vi "checkBeginEnemyPossesionAtOurField.vi"(8 "error in (no error)":errorcluster, 10 "Game":refnum<class "Game.lvclass">, 11 "EnemyPossessionAtOurFieldPlay in":refnum<class "EnemyPossessionAtOurFieldPlay.lvclass">) -> (0 "error out":errorcluster, 2 "Begin?":bool, 3 "EnemyPossessionAtOurFieldPlay out":refnum<class "EnemyPossessionAtOurFieldPlay.lvclass">)   [LabVIEW 2023, in "EnemyPossessionAtOurFieldPlay.lvclass"]
uses:
  EnemyPossessionAtOurFieldPlay.lvclass
  Game_class/Game.lvclass
  Team_class/OffensivePlay.ctl
  Referee_class/command_interpreted.ctl
  Events_class/Possession.ctl
  Game_class/Game.lvclass/Game.ctl
  Referee_class/Referee.lvclass/Referee.ctl
  Team_class/Team.lvclass/Team.ctl
  Parameters_class/Parameters.lvclass/Parameters.ctl
  Object_class/Object.lvclass/Object.ctl
  Ball_class/Ball.lvclass/Ball.ctl
  Events_class/Events.lvclass/Events.ctl
  Game_class/Read Referee.vi
  Game_class/Read EventsRef.vi
  Game_class/Read BallRef.vi
  Game_class/Read OffensiveTeam.vi
  Game_class/Read EnemyRef.vi
  Game_class/Read NewParameters.vi
  Game_class/Read FieldRef.vi
  Game_class/Read Parameters.lvclass.vi
  Parameters_class/Read BallVelToAbortPass.vi
  Team_class/Read RobotRef.vi
  Team_class/Read OffensivePlay.vi
  Object_class/Read x.vi
  Ball_class/Read velocityNorm.vi
  Events_class/Read id_touch.vi
  Events_class/Read touch.vi
  Referee_class/Read command_interpreted.vi
  <vilib>/Analysis/_algsub.llb/Vector Norm.vi
  <vilib>/Analysis/_algsub.llb/Real Vector Norm.vi
  Ally_class/Ally.lvclass
  C:/Users/ebert/Documents/codes/SSL/repo/SSL_AI/Team_class/Team.lvclass
  Enemy_class/Enemy.lvclass
  Ball_class/Ball.lvclass
  C:/Users/ebert/Documents/codes/SSL/repo/SSL_AI/Object_class/Object.lvclass
  Referee_class/Referee.lvclass
  Events_class/Events.lvclass
  Field_class/Field.lvclass
  Parameters_class/Parameters.lvclass
  Robot_class/Robot.lvclass
  Utilities_class/Utilities.lvclass
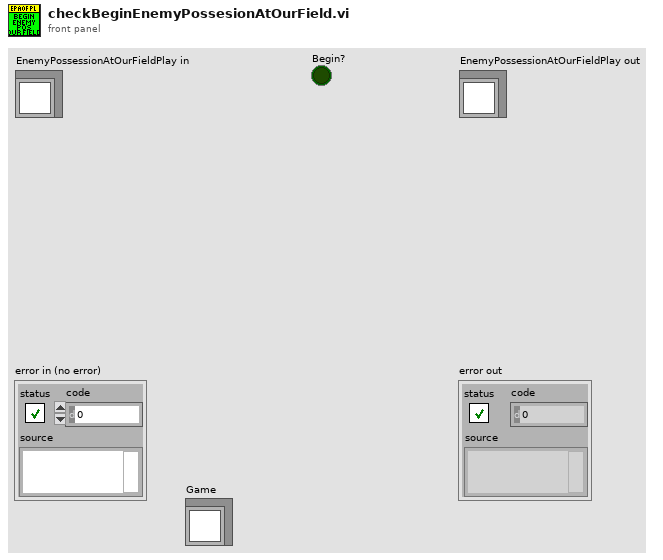
[diagram p1: front panel]
types:
  T1 = typedef "Events.lvclass/Possession.ctl" = enum16{"OurPossession", "TheirPossession", "Contended", "Loose"}
  T2 = typedef "OffensivePlay.ctl" = enum16{"5RobotsPassGamePlay", "5PreparePassGame", "5RobotsKeeperGame", "KeeperPassToStriker", "5RobotsNormalGamePlay", "PrepareKeeperPass", "ACBPass", "ABCPass", "PrepareTriplePass", "TableWithStriker", "TableWith2ndStrikerPlay", "PrepareDoublePass", "PrepareRollToPass", "SimplePass", "PreparePass", "PassToStriker", "BallOutOfField", "PassTo2ndStriker", "StopOffensive", "Prepare Penalty Enemy", "EnemyPossessionAtEnemyField", "EnemyPossesionAtOurField", "TestPlay", "PreparePenaltyAlly", "KickPenaltyAlly", "PrepareKickoffAlly", "PrepareKickoffEnemy", "IndirectEnemy", "DirectEnemy", "PreparePassInGame1", "NormalGame", "DirectKick", "Pass", "Halt", "Timeout", "PassPlay", "PenaltyEnemy"}
  T3 = typedef "command_interpreted.ctl" = enum16{"Goal Ally", "Goal Enemy", "Ball Placement Enemy", "Ball Placement Ally", "Normal Half Time", "Extra Time  Break", "Extra Half Time", "None", "Post Game", "PKA Normal Start", "Prepare Kickoff Ally", "PKE Normal Start", "Prepare Kickoff Enemy", "Force Start", "Halt", "Timeout", "Prepare Penalty Ally", "Prepare Penalty Enemy", "PPA NormalStart", "PPE Normal Start", "Indirect Free Ally", "Direct Free Enemy", "Direct Free Ally", "Indirect Free Enemy", "Stop"}
  T4 = typedef "NewParameters.ctl" = cluster{"PenaltyDistance":dbl, "DistanceAttackerToBackBall":dbl, "Division":enum16{"Div B", "Div A"}, "DistanceToAvoidyEnemyRobot":dbl, "BallPlacementDistance":dbl, "DisatanceBehindBallToStealBall":dbl, "MaxDistanceToPositionKickoff":dbl, "BlockEnemyTarget":bool, "MaxStopVAng":dbl, "DistanceMarkerToEnemy":dbl, "IgnoreDribblerContact":bool, "DistanceToBeginEnemyPosession":dbl, "GoToBallWhenEnemyNotMoving":bool, "EnemyDistanceToReduceVelocity":dbl, "TurnOnEnemyDistanceToReduceVelocity":bool, "EnemyDistanceToShootOutBall":dbl, "DefenseKickBall":bool, "MoreKickToGoal? (0-0.3)":dbl, "ChipKickInEnemyField":bool, "ShootOutRobotId":dbl, "FieldLenghtDenominatorInShootOut":dbl, "AdjustPositionInBallPlacement":bool, "PowerGodPass":dbl, "VelocityAbortEnemyPos":dbl, "MaxDistToBeginPass":dbl, "MinDistToBeginPass":dbl, "VelocityInDirects":dbl, "BadDribblerIDs":i32[], "NewKickToDistanceAroundBall":dbl, "PowerAvoidColisionMarker":dbl, "DistanceToAvoidColisionMarker":dbl, "AvoidBallKick":dbl, "DistanceTryKick":dbl, "SuicideKickDIstance":dbl, "FirstKickAtck":bool, "AdjustFirstKickDistance":dbl, "FirstKickDefense":bool, "AvoidAimLessKick":dbl, "DistanceToAvoidyEnemyShootRobot ":dbl, "NumberOfMarkers":dbl, "PotField":bool, "PIDLateral":bool, "MinDistanceFirstKickX":dbl, "MinDistanceFirstKickY":dbl, "FractionOfDistToTouchGround\nAfterChipKick":dbl, "FractionOfKickxWhen\nComposedWithKickz":dbl, "Style":T5, "MoveInTurnState":bool, "DistFromEnemyToConsider\nMoveInTurnState":dbl, "CascadePID":bool, "TurnAroundParameters":cluster{"Radius":dbl, "Multiplier":dbl, "ChordAngle":dbl}, "SafeDriveVel":dbl, "DistanceToGoToBackBall":dbl, "minDistanceToNotFinishEnemyPossession":dbl, "Probability to kick direct penalty (0 - 1)":dbl}
  T5 = typedef "Style.ctl" = enum16{"Insanity", "Offensive", "Defensive"}
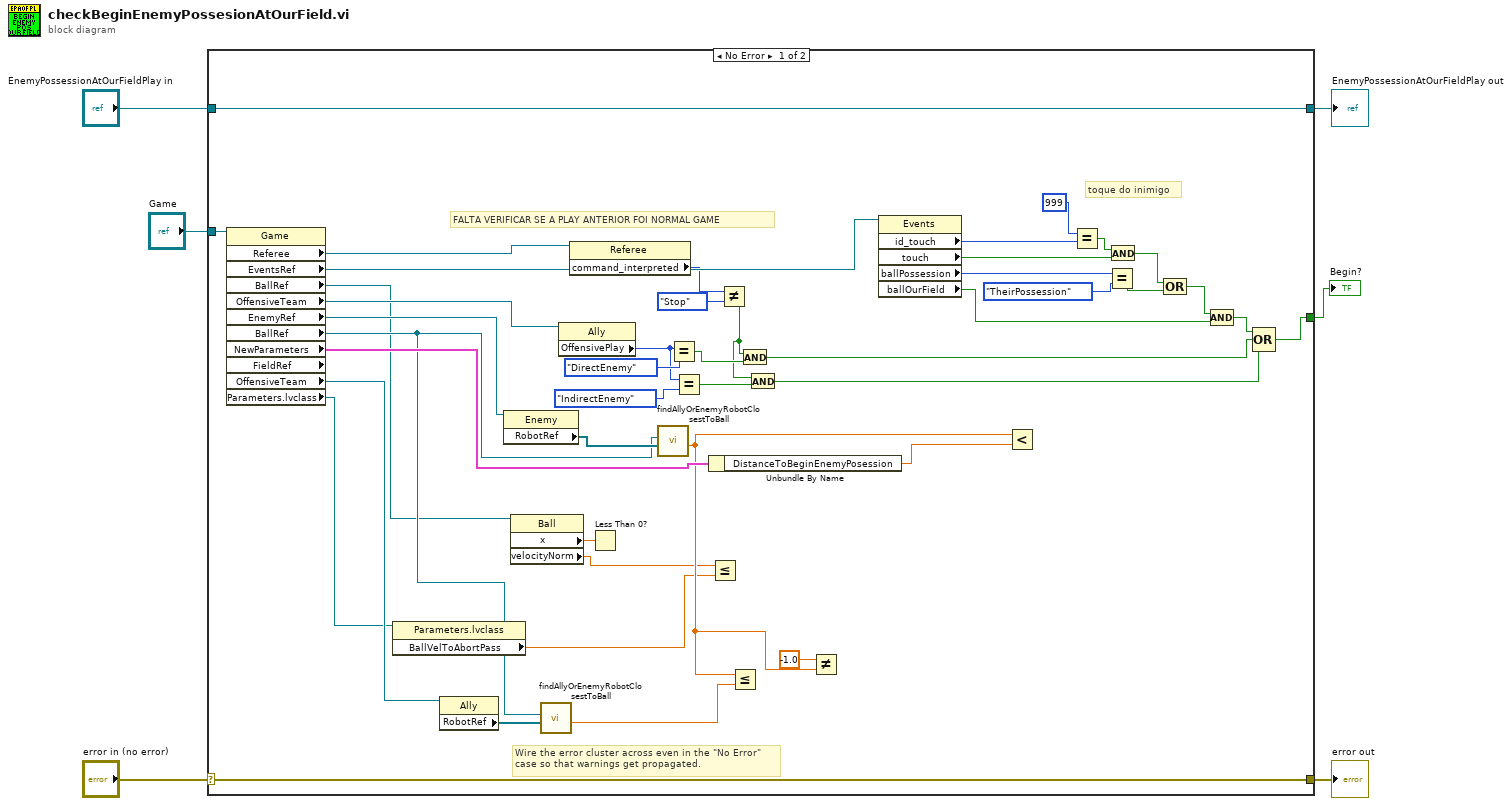
[diagram p0: block diagram]
diagram:
  n1 = case shown="No Error" "error in (no error)" {
    selector: "error in (no error)" -> [w48 w51]
    tunnel: [w48 w51] -> w5
    tunnel: [w49 w50] -> w3
    tunnel: "EnemyPossessionAtOurFieldPlay in" -> [w49 w50]
    tunnel: "Game" -> [w46 _]
    tunnel: [w7 _] -> w1
    frame No Error {
      # "toque do inimigo"
      # "FALTA VERIFICAR SE A PLAY ANTERIOR FOI NORMAL GAME"
      # "Wire the error cluster across even in the \"No Error\"\ncase so that warnings get propagated."
      n2 = property class="Game" props=["Referee", "EventsRef", "BallRef", "OffensiveTeam", "EnemyRef", "BallRef", "NewParameters", "FieldRef", "OffensiveTeam", "Parameters.lvclass"](reference=w46) -> ("Referee"=w42:refnum<class "Referee.lvclass">, "EventsRef"=w47:refnum<class "Events.lvclass">, "BallRef"=w21:refnum<class "Ball.lvclass">, "OffensiveTeam"=w45:refnum<class "Ally.lvclass">, "EnemyRef"=w31:refnum<class "Enemy.lvclass">, "BallRef"=w26:refnum<class "Ball.lvclass">, "NewParameters"=w30:T4, "OffensiveTeam"=w25:refnum<class "Ally.lvclass">, "Parameters.lvclass"=w19:refnum<class "Parameters.lvclass">)  [unwired: 1 in, 3 out]
      n3 = property class="Parameters.lvclass"(reference=w19) -> ("BallVelToAbortPass"=w18:dbl)  [unwired: 1 in, 2 out]
      n4 = property class="Ally"(reference=w25) -> ("RobotRef"=w24:refnum<class "Robot.lvclass">[])  [unwired: 1 in, 2 out]
      n5 = property class="Enemy"(reference=w31) -> ("RobotRef"=w27:refnum<class "Robot.lvclass">[])  [unwired: 1 in, 2 out]
      n6 = property class="Ball"(reference=w21) -> ("x"=w20:dbl, "velocityNorm"=w15:dbl)  [unwired: 1 in, 2 out]
      n7 = call "findAllyOrEnemyRobotClosestToBall.vi"("Ally/Enemy Robots"=w24, "Ball"=w26) -> ("Robot distance to ball"=w28:dbl)  [unwired: 5 in, 4 out]
      n8 = property class="Ally"(reference=w45) -> ("OffensivePlay"=w34:T2)  [unwired: 1 in, 2 out]
      n9 = property class="Referee"(reference=w42) -> ("command_interpreted"=w41:T3)  [unwired: 1 in, 2 out]
      n10 = Less Than 0?(x=w20) -> ()  [unwired: 1 out]
      n11 = call "findAllyOrEnemyRobotClosestToBall.vi"("Ally/Enemy Robots"=w27, "Ball"=w26) -> ("Robot distance to ball"=w23:dbl)  [unwired: 5 in, 4 out]
      n12 = Equal?(x=w34, y=OffensivePlay."DirectEnemy") -> (x = y?=w43:bool)
      n13 = Equal?(x=w34, y=OffensivePlay."IndirectEnemy") -> (x = y?=w33:bool)
      n14 = Unbundle By Name(w30) -> ("DistanceToBeginEnemyPosession"=w29:dbl)
      n15 = Less Or Equal?(x=w15, y=w18) -> ()  [unwired: 1 out]
      n16 = Not Equal?(x=w41, y=command_interpreted."Stop") -> (x != y?=w32:bool)
      n17 = Less Or Equal?(x=w23, y=w28) -> ()  [unwired: 1 out]
      n18 = And(x=w32, y=w43) -> (x .and. y?=w9:bool)
      n19 = And(x=w32, y=w33) -> (x .and. y?=w8:bool)
      n20 = Not Equal?(x=-1.0, y=w23) -> ()  [unwired: 1 out]
      n21 = property class="Events"(reference=w47) -> ("id_touch"=w38:i32, "touch"=w39:bool, "ballPossession"=w17:T1, "ballOurField"=w11:bool)  [unwired: 1 in, 2 out]
      n22 = Less?(x=w23, y=w29) -> ()  [unwired: 1 out]
      n23 = Equal?(x=999, y=w38) -> (x = y?=w36:bool)
      n24 = Equal?(x=w17, y=Possession."TheirPossession") -> (x = y?=w13:bool)
      n25 = And(x=w36, y=w39) -> (x .and. y?=w14:bool)
      n26 = Compound Arithmetic op=OR(w14, w13) -> (w12:bool)
      n27 = Compound Arithmetic op=AND(w12, w11) -> (w10:bool)
      n28 = Compound Arithmetic op=OR(w10, w9, w8) -> (w7:bool)
    }
    frame Error {
    }
  }
  "error out" <- w5
  "EnemyPossessionAtOurFieldPlay out" <- w3
  "Begin?" <- w1
